vi "Periodic Tasks.vi"(8 "error in":errorcluster) -> ()   [LabVIEW 2014]
doc: "This VI runs in parallel to other tasks. It can contain as many user-defined periodic loops as you need. These can carry out PID or other sorts of timed response."
uses:
  <vilib>/Rock Robotics/SystemInterfaces/Utilities/FPGA_UtilitiesLED Source.ctl
  <vilib>/Rock Robotics/SystemInterfaces/Utilities/FPGA_UtilitiesLED State.ctl
  Robot Global Data.vi
  <vilib>/Rock Robotics/SystemInterfaces/Typedef/FPGA_TypedefAnalogModule.ctl
  <vilib>/Rock Robotics/SystemInterfaces/AI/FPGA_AIChannel.ctl
  <vilib>/Rock Robotics/WPI/AnalogChannel/WPI_AnalogChannelDevRef.ctl
  <vilib>/gmath/NI_Gmath.lvlib
  <vilib>/Rock Robotics/SystemInterfaces/DIO/FPGA_DIOChannel.ctl
  <vilib>/Rock Robotics/SystemInterfaces/Typedef/FPGA_TypedefDigitalModule.ctl
  <vilib>/Rock Robotics/WPI/DigitalInput/WPI_DigitalInputDevRef.ctl
  Fire_Catapult_Enum.ctl
  <vilib>/Rock Robotics/WPI/SafetyOutput/WPI_SafetyOutputConfigMenu.ctl
  <vilib>/Rock Robotics/WPI/Solenoid/WPI_SolenoidSetEnum.vi
  <vilib>/Rock Robotics/WPI/Solenoid/WPI_SolenoidValue.ctl
panel:
  out "Catapult_Ready_To_Fire":bool
  in  "Tab Control":enum32{"Sensor_Config", "Override"}(tab)
  in  "Catapult_Switch_Channel":T1=enum."DIO 3"
  in  "CAM_Switch_Channel":T1=enum."DIO 5"
  in  "Invert_Catapult_Switch":bool
  in  "Invert_CAM_Switch":bool=TRUE
  in  "Mantis_Read_Channel":T2
  in  "Mantis_Read1_Voltage_Lookup":dbl[](array[numeric])=[4.38, 0.95] format="%_6g"
  in  "Mantis_Read1_Position_Lookup":dbl[](array[numeric])=[0.0, 100.0] format="%_6g"
  out "Mantis_Position_Raw_Voltage":dbl=2.023617081
  in  "Override_CAM_Switch_Enable":bool
  in  "Override_CAM_Switch_Val":bool=TRUE
  in  "Override_Catapult_Fully_Back_Enable":bool
  in  "Override_Mantis_Position_Enable":bool
  in  "Release_Override_Enable":bool
  in  "Winch_Override_Enable":bool
  in  "Winch_Override_Val":dbl
  in  "Override_Catapult_Fully_Back_Val":bool=TRUE
  in  "Override_Mantis_Position_Val":dbl=99.0
  in  "Release_Override_Val":dbl
  out "CAM_Switch_Value":bool
  out "Catapult_Switch_Value":bool=TRUE
  in  "Mantis_Arm_Firing_Position":dbl=90.0
  out "Firing_State":T3
  in  "Cataplut_Fire_Wait_Time":dbl=1.0 format="%#_13g"
  in  "Closed_Loop_Cycle_Time":dbl=0.01
  out "Catapult_Fully_Back":bool=TRUE
  out "Mantis_Position":dbl=68.69921046647232
  # "High State should be catapult retracted"
  # "Inputs"
  # "Outputs"
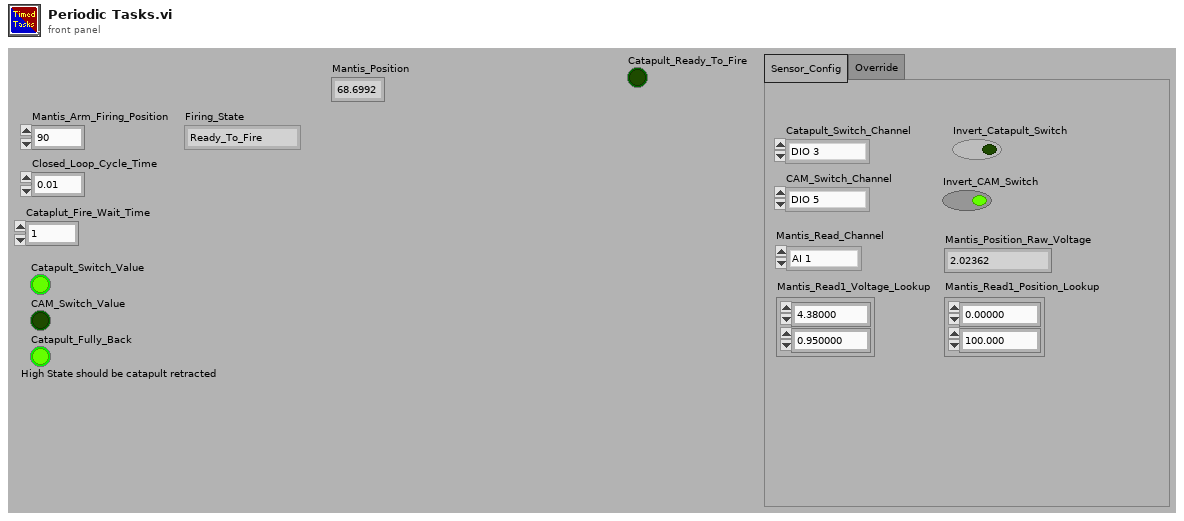
[diagram p1: front panel]
types:
  T1 = typedef "FPGA_DIOChannel.ctl" = enum8{"DIO 1", "DIO 2", "DIO 3", "DIO 4", "DIO 5", "DIO 6", "DIO 7", "DIO 8", "DIO 9", "DIO 10", "DIO 11", "DIO 12", "DIO 13", "DIO 14", "Invalid"}
  T2 = typedef "FPGA_AIChannel.ctl" = enum8{"AI 1", "AI 2", "AI 3", "AI 4", "AI 5", "AI 6", "AI 7", "AI 8", "Invalid"}
  T3 = typedef "Fire_Catapult_Enum.ctl" = enum16{"Ready_To_Fire", "Operate_Release", "Wait_For_Catapult_To_Finish_Fire", "Engage_Winch", "Halt_Winch"}
  T4 = typedef "WPI_CompressorDevRef.ctl" = cluster{"DevStatus":errorcluster, "DigitalInputDevRef":T5, "RelayDevRef":T7}
  T5 = typedef "WPI_DigitalInputDevRef.ctl" = cluster{"DevStatus":errorcluster, "DIO Channel":T1, "Digital Module":T6}
  T6 = typedef "FPGA_TypedefDigitalModule.ctl" = enum16{"Digital Module 1", "Digital Module 2"}
  T7 = typedef "WPI_RelayDevRef.ctl" = cluster{"DevStatus":errorcluster, "Relay Channel":T8, "Digital Module":T6, "Relay Direction":T9}
  T8 = typedef "FPGA_DIORelayChannel.ctl" = enum8{"Relay 1", "Relay 2", "Relay 3", "Relay 4", "Relay 5", "Relay 6", "Relay 7", "Relay 8", "Invalid"}
  T9 = typedef "WPI_RelayDirection.ctl" = enum16{"Both directions", "Forward only", "Reverse only"}
  T10 = typedef "WPI_JoystickDevRef.ctl" = cluster{"Device":T11}
  T11 = typedef "WPI_JoystickDeviceEnum.ctl" = enum16{"USB 0", "USB 1", "USB 2", "USB 3", "USB 4", "USB 5"}
  T12 = typedef "WPI_RobotDriveDevRef.ctl" = cluster{"DevStatus":errorcluster, "Motors[]":T13[], "Square Inputs":bool, "Max Output":dbl}
  T13 = typedef "WPI_MotorControlDeviceRef.ctl" = cluster{"DeviceStatus":errorcluster, "Type":enum16{"PWM", "CAN"}, "PWM":cluster{"Digital Module":T6, "PWM Channel":T14, "DeadBand":T15}, "CAN":cluster{"Device Number":u8, "Control Mode":T16, "Semaphore":T17, "Max Vout":dbl}, "Invert":bool, "TransformRef":T18, "InvTransformRef":T18}
  T14 = typedef "FPGA_DIOPWMChannel.ctl" = enum8{"PWM 1", "PWM 2", "PWM 3", "PWM 4", "PWM 5", "PWM 6", "PWM 7", "PWM 8", "PWM 9", "PWM 10", "Invalid"}
  T15 = typedef "WPI_PWMDeadband.ctl" = cluster{"Name":string, "maxPositivePwm":i32, "minPositivePwm":i32, "centerPwm":i32, "maxNegativePwm":i32, "minNegativePwm":i32, "angularRange":u16}
  T16 = typedef "WPI_CANJaguar_ControlMode.ctl" = enum8{"Percent VBus", "Current", "Speed", "Position", "Voltage"}
  T17 = typedef "Semaphore RefNum" = refnum<k1>
  T18 = typedef "WPI_PWMTransform_ConPane.ctl" = refnum<vi>
  T19 = cluster{"JoystickDevRef":T10, "RobotDriveDevRef":T12}
  T20 = typedef "FPGA_TypedefAnalogModule.ctl" = enum16{"Analog Module 1", "Analog Module 2"}
  T21 = typedef "WPI_AnalogChannelDevRef.ctl" = cluster{"DevStatus":errorcluster, "Analog Module":T20, "Analog Channel":T2}
  T22 = typedef "WPI_SolenoidValue.ctl" = enum16{"Off", "On", "Forward", "Reverse"}
  T23 = typedef "WPI_SafetyOutputConfigMenu.ctl" = enum16{"Enable", "Disable"}
  T24 = typedef "WPI_SolenoidDevRef.ctl" = cluster{"DevStatus":errorcluster, "Solenoid Module":T25, "Forward Solenoid Channel":T26, "Reverse Solenoid Channel":T26}
  T25 = typedef "FPGA_TypedefSolenoidModule.ctl" = enum16{"Solenoid Module 1", "Solenoid Module 2"}
  T26 = typedef "WPI_SolenoidChannel.ctl" = enum8{"Solenoid 1", "Solenoid 2", "Solenoid 3", "Solenoid 4", "Solenoid 5", "Solenoid 6", "Solenoid 7", "Solenoid 8", "Invalid"}
  T27 = typedef "FPGA_UtilitiesLED State.ctl" = enum16{"Off", "On", "Toggle"}
  T28 = typedef "FPGA_UtilitiesLED Source.ctl" = enum16{"User LED", "FPGA LED"}
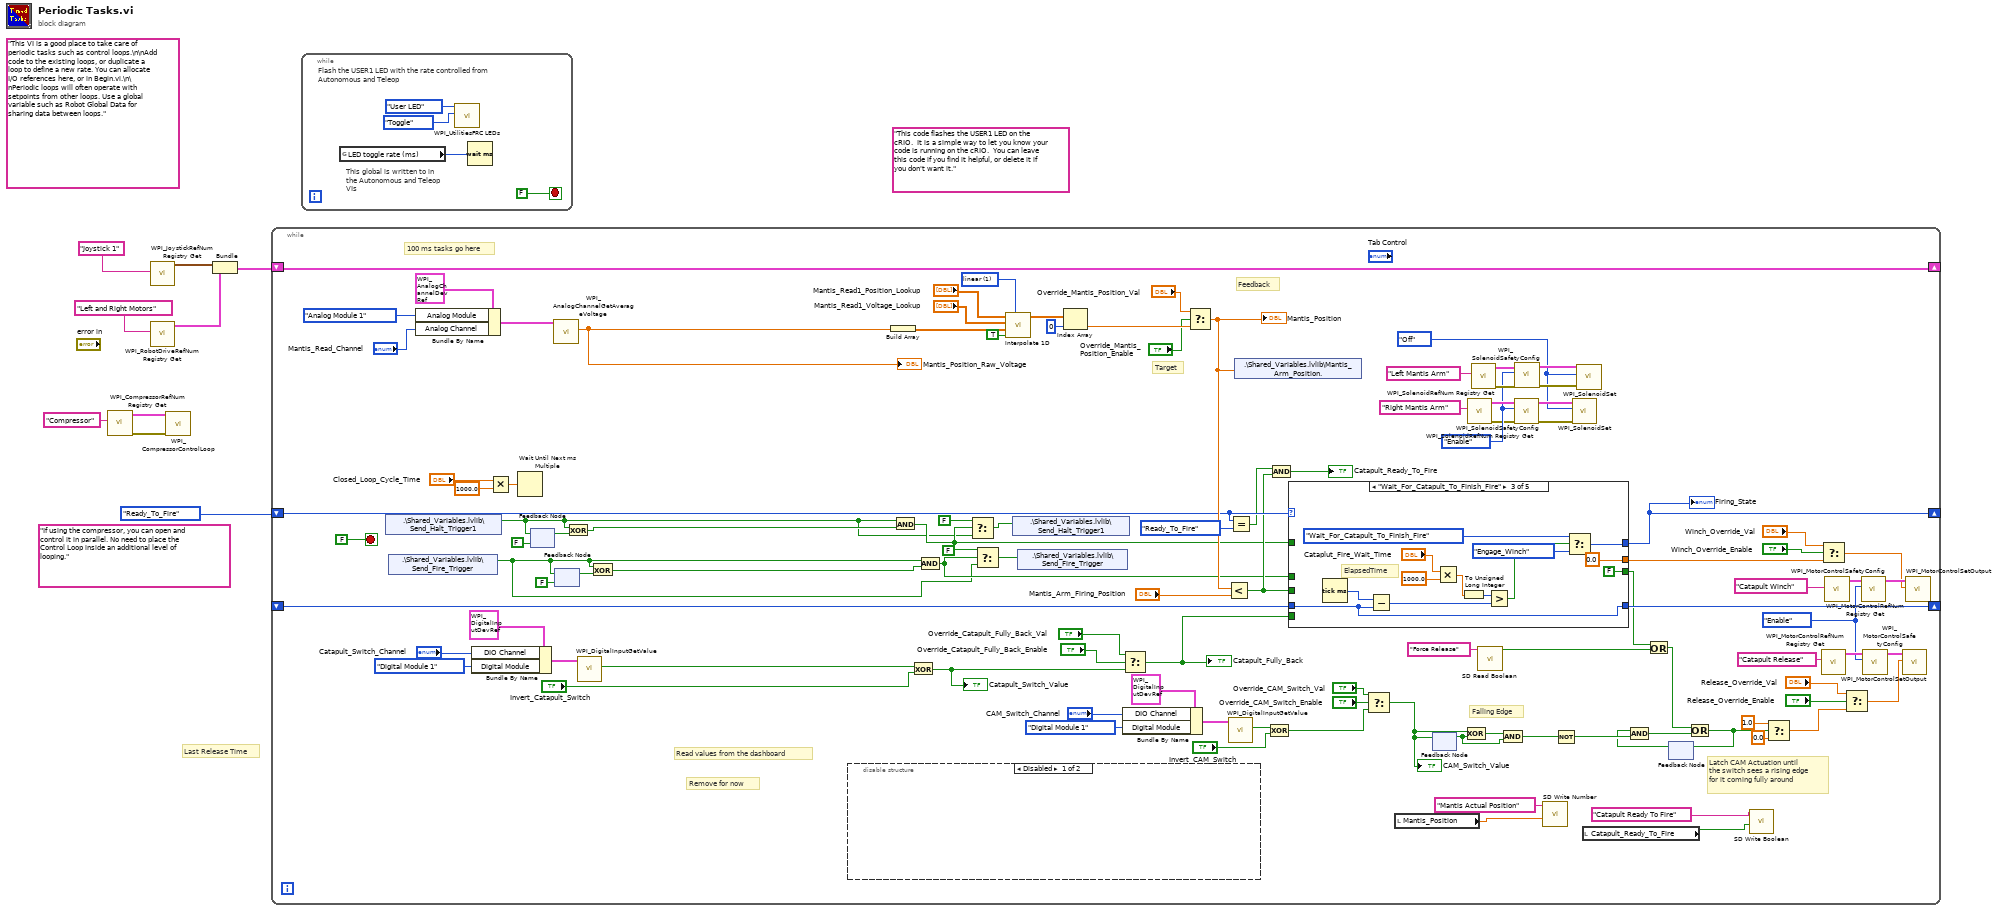
[diagram p0: block diagram]
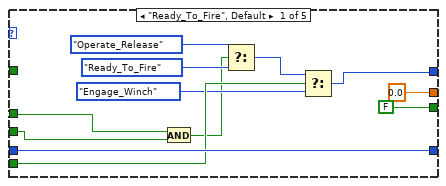
[diagram p3: hidden frame]
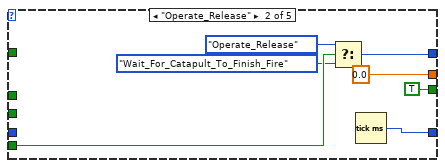
[diagram p4: hidden frame]
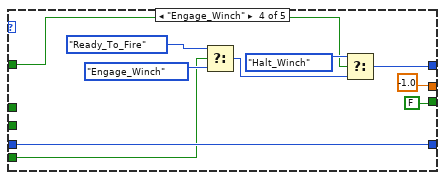
[diagram p5: hidden frame]
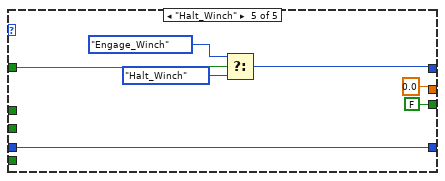
[diagram p6: hidden frame]
diagram:
  (unwired) "If using the compressor, you can open and control it in parallel. No need to place the Control Loop inside an additional level of looping."
  (unwired) "This code flashes the USER1 LED on the cRIO.  It is a simple way to let you know your code is running on the cRIO.  You can leave this code if you find it helpful, or delete it if you don't want it."
  (unwired) "This VI is a good place to take care of periodic tasks such as control loops.\n\nAdd code to the existing loops, or duplicate a loop to define a new rate. You can allocate I/O references here, or in Begin.vi.\n\nPeriodic loops will often operate with setpoints from other loops. Use a global variable such as Robot Global Data for sharing data between loops."
  # "Last Release Time"
  n1 = call <vilib>:"WPI_CompressorRefNum Registry Get.vi"("refnum name"="Compressor") -> ("error out"=w2:errorcluster, "CompressorDevRef"=w3:T4)  [unwired: 9 in]
  n2 = call <vilib>:"WPI_JoystickRefNum Registry Get.vi"("refnum name"="Joystick 1") -> ("JoystickDevRef"=w7:T10)  [unwired: 1 in, 9 out]
  n3 = call <vilib>:"WPI_RobotDriveRefNum Registry Get.vi"("refnum name"="Left and Right Motors") -> ("RobotDriveDevRef"=w6:T12)  [unwired: 1 in, 9 out]
  n4 = call <vilib>:"WPI_CompressorControlLoop.vi"("error in (no error)"=w2, "CompressorDevRef"=w3) -> ()  [unwired: 10 in]
  n5 = Bundle("JoystickDevRef"=w7, "RobotDriveDevRef"=w6) -> (w5:T19)  [unwired: 1 out]
  n6 = while {
    shift-right: [w116] -> _
    shift-left: w5 -> [w116]
    shift-right: [w85] -> _
    shift-left: Fire_Catapult_Enum."Ready_To_Fire" -> [w43]
    shift-right: [w83] -> _
    shift-left: _ -> [w84]
    stop <- FALSE stop-if-true
    w10 = WPI_SolenoidValue."Off" ("Value")
    w51 = WPI_SafetyOutputConfigMenu."Enable" ("mode")
    w14 = WPI_SafetyOutputConfigMenu."Enable" ("mode")
    w106 = 1 items=["nearest", "linear", "spline", "cubic Hermite", "Lagrange"] ("method")
    # "Remove for now"
    # "Read values from the dashboard"
    # "Latch CAM Actuation until\nthe switch sees a rising edge\nfor it coming fully around"
    # "Falling Edge"
    # "Feedback"
    # "Target"
    # "100 ms tasks go here"
    n7 = shared-variable ".\\Shared_Variables.lvlib\\Send_Halt_Trigger1"() -> (w26:bool)  [unwired: 1 in, 1 out]
    n8 = shared-variable ".\\Shared_Variables.lvlib\\Send_Fire_Trigger"() -> (w31:bool)  [unwired: 1 in, 1 out]
    n9 = Bundle By Name(cluster=T21 {"DevStatus"={"status"=FALSE, "code"=0, "source"=""}, "Analog Module"=enum."Analog Module 1", "Analog Channel"=enum."AI 1"} ("AIDeviceRef"), "Analog Module"=FPGA_TypedefAnalogModule."Analog Module 1", "Analog Channel"="Mantis_Read_Channel") -> (w114:T21)
    n10 = Bundle By Name(cluster=T5 {"DevStatus"={"status"=FALSE, "code"=0, "source"=""}, "DIO Channel"=enum."DIO 1", "Digital Module"=enum."Digital Module 1"} ("DigitalInputDevRef"), "DIO Channel"="Catapult_Switch_Channel", "Digital Module"=FPGA_TypedefDigitalModule."Digital Module 1") -> (w102:T5)
    n11 = Multiply(x="Closed_Loop_Cycle_Time", y=1000.0) -> (x*y=w88:dbl)
    n12 = Wait Until Next ms Multiple(millisecond multiple=w88) -> ()  [unwired: 1 out]
    n13 = feedback #1(FALSE ("Boolean")) -> (w53:bool)
    n14 = feedback-in #1(w26) -> ()
    n15 = call <vilib>:"WPI_AnalogChannelGetAverageVoltage.vi"("AIDeviceRef"=w114) -> ("Voltage"=w111:dbl)  [unwired: 8 in, 2 out]
    "Mantis_Position_Raw_Voltage" <- w111
    n16 = feedback #2(FALSE ("Boolean")) -> (w36:bool)
    n17 = feedback-in #2(w31) -> ()
    n18 = Exclusive Or(1:w53, 2:w26) -> (0:w52:bool)
    n19 = call <vilib>:"WPI_DigitalInputGetValue.vi"("DigitalInputDevRef"=w102) -> ("Value"=w99:bool)  [unwired: 8 in, 2 out]
    n20 = Exclusive Or(1:w36, 2:w31) -> (0:w35:bool)
    n21 = disable-structure shown="Disabled" {
      frame Disabled {
      }
      frame Enabled {
      }
    }
    n22 = Build Array(w111) -> (w110:dbl[])
    n23 = And(x=w26, y=w52) -> (x .and. y?=w27:bool)
    n24 = Exclusive Or(1:"Invert_Catapult_Switch", 2:w99) -> (0:w93:bool)
    "Catapult_Switch_Value" <- w93
    n25 = And(x=w31, y=w35) -> (x .and. y?=w33:bool)
    n26 = Select(t=FALSE ("Boolean"), s=w27, f=w26) -> (s? t:f=w28:bool)
    n27 = Select(t=FALSE ("Boolean"), s=w33, f=w31) -> (s? t:f=w30:bool)
    n28 = call <vilib>:"Interpolate 1D.vi"("method"=w106, "X is monotonic"=TRUE, "xi"=w110, "X"="Mantis_Read1_Voltage_Lookup", "Y"="Mantis_Read1_Position_Lookup") -> ("yi"=w107:dbl[])  [unwired: 4 in, 2 out]
    n29 = shared-variable ".\\Shared_Variables.lvlib\\Send_Halt_Trigger1"(w28) -> ()  [unwired: 1 in, 1 out]
    n30 = shared-variable ".\\Shared_Variables.lvlib\\Send_Fire_Trigger"(w30) -> ()  [unwired: 1 in, 1 out]
    n31 = Index Array(array=w107, index=0) -> (element=w97:dbl)
    n32 = Select(t="Override_Catapult_Fully_Back_Val", s="Override_Catapult_Fully_Back_Enable", f=w93) -> (s? t:f=w23:bool)
    "Catapult_Fully_Back" <- w23
    n33 = Bundle By Name(cluster=T5 {"DevStatus"={"status"=FALSE, "code"=0, "source"=""}, "DIO Channel"=enum."DIO 1", "Digital Module"=enum."Digital Module 1"} ("DigitalInputDevRef"), "DIO Channel"="CAM_Switch_Channel", "Digital Module"=FPGA_TypedefDigitalModule."Digital Module 1") -> (w73:T5)
    n34 = Select(t="Override_Mantis_Position_Val", s="Override_Mantis_Position_Enable", f=w97) -> (s? t:f=w45:dbl)
    "Mantis_Position" <- w45
    n35 = Less?(x=w45, y="Mantis_Arm_Firing_Position") -> (x < y?=w41:bool)
    n36 = call <vilib>:"WPI_DigitalInputGetValue.vi"("DigitalInputDevRef"=w73) -> ("Value"=w71:bool)  [unwired: 8 in, 2 out]
    n37 = Equal?(x=w43, y=Fire_Catapult_Enum."Ready_To_Fire") -> (x = y?=w40:bool)
    n38 = shared-variable ".\\Shared_Variables.lvlib\\Mantis_Arm_Position."(w45) -> ()  [unwired: 1 in, 1 out]
    n39 = Exclusive Or(1:"Invert_CAM_Switch", 2:w71) -> (0:w47:bool)
    n40 = And(x=w40, y=w41) -> (x .and. y?=→"Catapult_Ready_To_Fire":bool)
    n41 = case shown="\"Wait_For_Catapult_To_Finish_Fire\"" w43 {
      tunnel: [w125 w134 w142 w152 w161] -> w85
      tunnel: w23 -> [w124 w136 _ w151 _]
      tunnel: [0.0 0.0 0.0 -1.0 0.0] -> w61
      tunnel: [w127 w132 w140 w159 w164] -> w83
      tunnel: w84 -> [w127 _ w140 w159 w164]
      tunnel: [FALSE TRUE FALSE FALSE FALSE] -> w58
      tunnel: w33 -> [w118 _ _ _ _]
      tunnel: w27 -> [_ _ _ w150 w163]
      tunnel: w41 -> [w119 _ _ _ _]
      frame "Ready_To_Fire", Default {
        n42 = And(x=w118, y=w119) -> (x .and. y?=w121:bool)
        n43 = Select(t=Fire_Catapult_Enum."Operate_Release", s=w121, f=Fire_Catapult_Enum."Ready_To_Fire") -> (s? t:f=w126:T3)
        n44 = Select(t=w126, s=w124, f=Fire_Catapult_Enum."Engage_Winch") -> (s? t:f=w125:T3)
      }
      frame "Operate_Release" {
        n45 = Select(t=Fire_Catapult_Enum."Operate_Release", s=w136, f=Fire_Catapult_Enum."Wait_For_Catapult_To_Finish_Fire") -> (s? t:f=w134:T3)
        n46 = Tick Count (ms)() -> (millisecond timer value=w132:u32)
      }
      frame "Wait_For_Catapult_To_Finish_Fire" {
        # "ElapsedTime"
        n47 = Tick Count (ms)() -> (millisecond timer value=w149:u32)
        n48 = Subtract(x=w149, y=w140) -> (x-y=w146:u32)
        n49 = Multiply(x="Cataplut_Fire_Wait_Time", y=1000.0) -> (x*y=w144:dbl)
        n50 = To Unsigned Long Integer(number=w144) -> (unsigned 32bit integer=w145:u32)
        n51 = Greater?(x=w145, y=w146) -> (0:w141:bool)
        n52 = Select(t=Fire_Catapult_Enum."Wait_For_Catapult_To_Finish_Fire", s=w141, f=Fire_Catapult_Enum."Engage_Winch") -> (s? t:f=w142:T3)
      }
      frame "Engage_Winch" {
        n53 = Select(t=Fire_Catapult_Enum."Ready_To_Fire", s=w151, f=Fire_Catapult_Enum."Engage_Winch") -> (s? t:f=w153:T3)
        n54 = Select(t=Fire_Catapult_Enum."Halt_Winch" ("f"), s=w150, f=w153) -> (s? t:f=w152:T3)
      }
      frame "Halt_Winch" {
        n55 = Select(t=Fire_Catapult_Enum."Engage_Winch" ("f"), s=w163, f=Fire_Catapult_Enum."Halt_Winch") -> (s? t:f=w161:T3)
      }
    }
    "Firing_State" <- w85
    n56 = Select(t="Override_CAM_Switch_Val", s="Override_CAM_Switch_Enable", f=w47) -> (s? t:f=w46:bool)
    "CAM_Switch_Value" <- w46
    n57 = local read "Mantis_Position"() -> (w37:dbl)
    n58 = feedback-in #3(w46) -> ()
    n59 = feedback #3() -> (w54:bool)  [unwired: 1 in]
    n60 = Exclusive Or(1:w54, 2:w46) -> (0:w55:bool)
    n61 = call <vilib>:"WPI_SolenoidRefNum Registry Get.vi"("refnum name"="Right Mantis Arm") -> ("error out"=w11:errorcluster, "SolenoidDevRef"=w20:T24)  [unwired: 9 in]
    n62 = call <vilib>:"WPI_SolenoidRefNum Registry Get.vi"("refnum name"="Left Mantis Arm") -> ("error out"=w17:errorcluster, "SolenoidDevRef"=w16:T24)  [unwired: 9 in]
    n63 = call <vilib>:"SD Read Boolean.vi"("Name"="Force Release") -> ("Boolean"=w21:bool)  [unwired: 8 in, 2 out]
    n64 = And(x=w55, y=w54) -> (x .and. y?=w56:bool)
    n65 = call <vilib>:"WPI_SolenoidSafetyConfig.vi"("error in (no error)"=w11, "mode"=w14, "SolenoidDevRef"=w20) -> ("error out"=w12:errorcluster, "SolenoidDevRef 2"=w19:T24)  [unwired: 7 in]
    n66 = call <vilib>:"WPI_SolenoidSafetyConfig.vi"("error in (no error)"=w17, "mode"=w14, "SolenoidDevRef"=w16) -> ("error out"=w13:errorcluster, "SolenoidDevRef 2"=w15:T24)  [unwired: 7 in]
    n67 = call <vilib>:"SD Write Number.vi"("Numeric"=w37, "Name"="Mantis Actual Position") -> ()  [unwired: 8 in, 2 out]
    n68 = Not(x=w56) -> (.not. x?=w69:bool)
    n69 = call-poly <vilib>:"WPI_SolenoidSet.vi"("error in (no error)"=w12, "Value"=w10, "SolenoidDevRef"=w19) -> ()  [unwired: 7 in, 2 out]
    n70 = call-poly <vilib>:"WPI_SolenoidSet.vi"("error in (no error)"=w13, "Value"=w10, "SolenoidDevRef"=w15) -> ()  [unwired: 7 in, 2 out]
    n71 = local read "Catapult_Ready_To_Fire"() -> (w24:bool)
    n72 = Or(x=w58, y=w21) -> (x .or. y?=w57:bool)
    n73 = feedback #4() -> (w67:bool)  [unwired: 1 in]
    n74 = And(x=w67, y=w69) -> (x .and. y?=w68:bool)
    n75 = Or(x=w57, y=w68) -> (x .or. y?=w66:bool)
    n76 = feedback-in #4(w66) -> ()
    n77 = call <vilib>:"SD Write Boolean.vi"("Boolean"=w24, "Name"="Catapult Ready To Fire") -> ()  [unwired: 8 in, 2 out]
    n78 = Select(t=1.0, s=w66, f=0.0) -> (s? t:f=w63:dbl)
    n79 = Select(t="Winch_Override_Val", s="Winch_Override_Enable", f=w61) -> (s? t:f=w59:dbl)
    n80 = call <vilib>:"WPI_MotorControlRefNum Registry Get.vi"("refnum name"="Catapult Release") -> ("MotorControlDevRef"=w80:T13)  [unwired: 9 in, 1 out]
    n81 = call <vilib>:"WPI_MotorControlRefNum Registry Get.vi"("refnum name"="Catapult Winch") -> ("MotorControlDevRef"=w82:T13)  [unwired: 9 in, 1 out]
    n82 = Select(t="Release_Override_Val", s="Release_Override_Enable", f=w63) -> (s? t:f=w78:dbl)
    n83 = call <vilib>:"WPI_MotorControlSafetyConfig.vi"("mode"=w51, "MotorControlDevRef"=w82) -> ("MotorControlDevRef"=w81:T13)  [unwired: 8 in, 1 out]
    n84 = call <vilib>:"WPI_MotorControlSafetyConfig.vi"("mode"=w51, "MotorControlDevRef"=w80) -> ("MotorControlDevRef"=w79:T13)  [unwired: 8 in, 1 out]
    n85 = call <vilib>:"WPI_MotorControlSetOutput.vi"("Output"=w78, "MotorControlDevRef"=w79) -> ()  [unwired: 7 in, 3 out]
    n86 = call <vilib>:"WPI_MotorControlSetOutput.vi"("Output"=w59, "MotorControlDevRef"=w81) -> ()  [unwired: 7 in, 3 out]
  }
  n87 = while {
    stop <- FALSE stop-if-true
    # "This global is written to in the Autonomous and Teleop VIs"
    # "Flash the USER1 LED with the rate controlled from Autonomous and Teleop"
    n88 = global read "Robot Global Data.vi" "LED toggle rate (ms)"() -> (w167:u32)
    n89 = call <vilib>:"WPI_UtilitiesFRC LEDs.vi"("State"=FPGA_UtilitiesLED_State."Toggle", "LED Type"=FPGA_UtilitiesLED_Source."User LED") -> ()  [unwired: 1 in, 9 out]
    n90 = Wait (ms)(milliseconds to wait=w167) -> ()  [unwired: 1 out]
  }
